vi "IFA300CommandDescriptors.vi"(4 "IFACommand":T2="ReadErrorQueue") -> (0 "Error":bool, 1 "CommandDescriptorOutput":T1={"Command"="ReadErrorQueue", "Mnemonic"="*STAT?", "ActionPath"=["PassCommand", "Communicate", "ParseError", "Done"]})   [LabVIEW 2012]
uses:
  IFA300Command.ctl
  IFA300CommandDescriptor.ctl
  IFA300CommandPhases.ctl
panel:
  in  "CommandDescriptorArray":T1[](array[typedef])=[{"Command"="Reset", "Mnemonic"="*RST", "ActionPath"=["PassCommand", "Communicate", "Done"]}, {"Command"="Version", "Mnemonic"="*IDN?", "ActionPath"=["PassCommand", "Communicate", "Done"]}, {"Command"="ReadErrorQueue", "Mnemonic"="*STAT?", "ActionPath"=["PassCommand", "Communicate", "ParseError", "Done"]}, {"Command"="CountChannels", "Mnemonic"="INST:CNUM?", "ActionPath"=["PassCommand", "Communicate", "ParseNumber", "Done"]}, {"Command"="CheckDaisyChain", "Mnemonic"="INST:IFA? ", "ActionPath"=["PassCommand", "Communicate", "ParseNumber", "Done"]}, {"Command"="MeasureCableResistance", "Mnemonic"="MEAS:RCBL", "ActionPath"=["AddressCommand", "Communicate", "Done"]}, {"Command"="ReadbackCableResistance", "Mnemonic"="READ:RCBL?", "ActionPath"=["PassCommand", "Communicate", "ParseNumber", "Done"]}, {"Command"="MeasureColdResistance", "Mnemonic"="MEAS:RMES", "ActionPath"=["AddressCommand", "Communicate", "Done"]}, {"Command"="ReadbackColdResistance", "Mnemonic"="READ:RMES?", "ActionPath"=["PassCommand", "Communicate", "ParseNumber", "Done"]}, {"Command"="SelectChannel", "Mnemonic"="INST:NSEL", "ActionPath"=["AddressCommand", "Communicate", "Done"]}, {"Command"="MonitorChannel", "Mnemonic"="OUTP:VOLT", "ActionPath"=["AddressCommand", "Communicate", "Done"]}, {"Command"="Complete?", "Mnemonic"="*OPC?", "ActionPath"=["PassCommand", "Communicate", "ParseNumber", "Done"]}, {"Command"="SetHotResistance", "Mnemonic"="CONF:ROP", "ActionPath"=["AppendVariable", "Communicate", "Done"]}, {"Command"="ReadHotResistance", "Mnemonic"="READ:ROP?", "ActionPath"=["PassCommand", "Communicate", "ParseNumber", "Done"]}, {"Command"="ReadAnemometerType", "Mnemonic"="READ:ANEM?", "ActionPath"=["PassCommand", "Communicate", "Done"]}, {"Command"="SetProbeType", "Mnemonic"="CONF:PROB", "ActionPath"=["AppendVariable", "Communicate", "Done"]}, {"Command"="ReadProbeType", "Mnemonic"="READ:PROB?", "ActionPath"=["PassCommand", "Communicate", "Done"]}, {"Command"="SetHighPowerBridgeOn", "Mnemonic"="CONF:HPWR", "ActionPath"=["AppendVariable", "Communicate", "Done"]}, {"Command"="SetCableLength", "Mnemonic"="CONF:CABL", "ActionPath"=["AppendVariable", "Communicate", "Done"]}, {"Command"="RunMode", "Mnemonic"="INIT:STAR", "ActionPath"=["AddressCommand", "Communicate", "Done"]}, {"Command"="StandbyMode", "Mnemonic"="INIT:STOP", "ActionPath"=["AddressCommand", "Communicate", "Done"]}, {"Command"="GetMode", "Mnemonic"="INIT:STAT?", "ActionPath"=["AddressCommand", "Communicate", "ParseNumber", "Done"]}, {"Command"="StandbyAll", "Mnemonic"="ABOR", "ActionPath"=["PassCommand", "Communicate", "Done"]}, {"Command"="OverrideOverheat", "Mnemonic"="CONF:OVHT", "ActionPath"=["AppendVariable", "Communicate", "Done"]}, {"Command"="ReadOverheat", "Mnemonic"="READ:OVHT", "ActionPath"=["PassCommand", "Communicate", "ParseNumber", "Done"]}, {"Command"="ReadBridgeVoltage", "Mnemonic"="READ:BDGV?", "ActionPath"=["PassCommand", "Communicate", "ParseNumber", "Done"]}, {"Command"="SetGain", "Mnemonic"="CONF:GAIN", "ActionPath"=["AppendVariable", "Communicate", "Done"]}, {"Command"="ReadGain", "Mnemonic"="READ:GAIN?", "ActionPath"=["PassCommand", "Communicate", "ParseNumber", "Done"]}, {"Command"="SetOffset", "Mnemonic"="CONF:OFFS", "ActionPath"=["AppendVariable", "Communicate", "Done"]}, {"Command"="ReadOffset", "Mnemonic"="READ:OFFS?", "ActionPath"=["PassCommand", "Communicate", "ParseNumber", "Done"]}, {"Command"="SetLowpassFilter", "Mnemonic"="OUTP:FILT", "ActionPath"=["AppendVariable", "Communicate", "Done"]}, {"Command"="SetHighpassFilter", "Mnemonic"="OUTP:HPAS", "ActionPath"=["AppendVariable", "Communicate", "Done"]}, {"Command"="SetThermocoupleRange", "Mnemonic"="CONF:TEMP", "ActionPath"=["AppendVariable", "Communicate", "Done"]}, {"Command"="MeasureTemperature", "Mnemonic"="MEAS:TEMP", "ActionPath"=["PassCommand", "Communicate", "Done"]}, {"Command"="ReadTemperature", "Mnemonic"="READ:TEMP?", "ActionPath"=["PassCommand", "Communicate", "ParseNumber", "Done"]}, {"Command"="SqWaveFreq", "Mnemonic"="TEST:FREQ", "ActionPath"=["AppendVariable", "Communicate", "Done"]}, {"Command"="SqWaveVolts", "Mnemonic"="TEST:VOLT", "ActionPath"=["AppendVariable", "Communicate", "Done"]}]
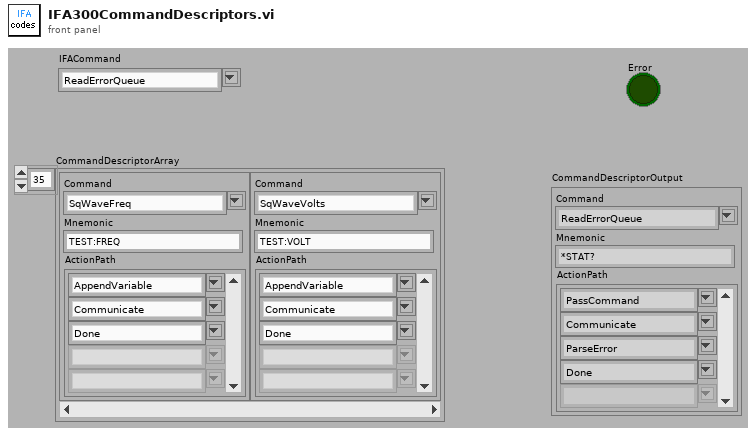
[diagram p1: front panel]
types:
  T1 = typedef "IFA300CommandDescriptor.ctl" = cluster{"Command":T2, "Mnemonic":string, "ActionPath":T3[]}
  T2 = typedef "IFA300Command.ctl" = string
  T3 = typedef "IFA300CommandPhases.ctl" = string
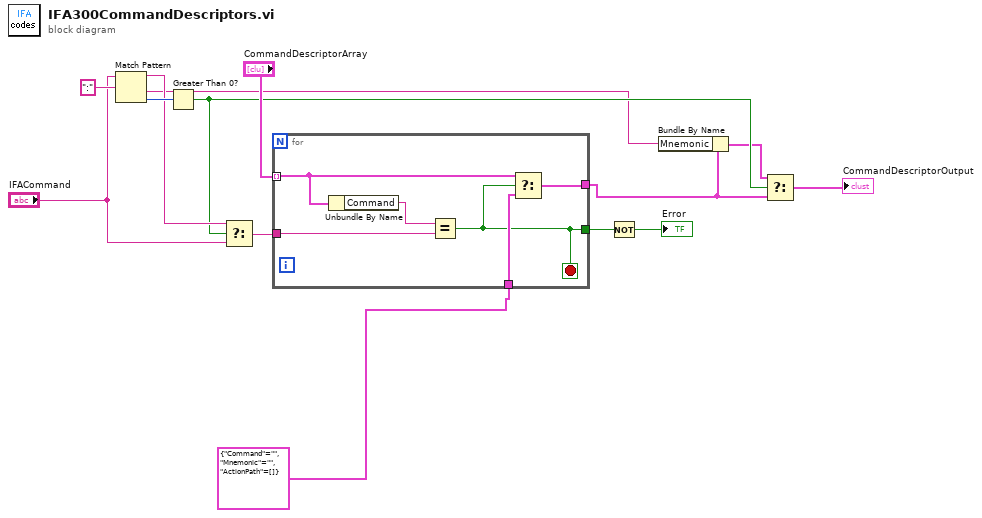
[diagram p0: block diagram]
diagram:
  n1 = Match Pattern(string="IFACommand", regular expression=":") -> (before substring=w7:T2, after substring=w2:T2, offset past match=w10:i32)  [unwired: 2 out]
  n2 = Greater Than 0?(x=w10) -> (x > 0?=w5:bool)
  n3 = Select(t=w7, s=w5, f="IFACommand") -> (s? t:f=w9:T2)
  n4 = for {
    tunnel: "CommandDescriptorArray" -> [w17] mode=indexing
    tunnel: w9 -> [w19]
    tunnel: [w18] -> w4
    tunnel: T1 {"Command"="", "Mnemonic"="", "ActionPath"=[]} ("s? t:f") -> [w16]
    tunnel: [w15] -> w13
    stop <- w15 stop-if-true
    n5 = Unbundle By Name(w17) -> ("Command"=w20:T2)
    n6 = Equal?(x=w20, y=w19) -> (x = y?=w15:bool)
    n7 = Select(t=w17, s=w15, f=w16) -> (s? t:f=w18:T1)
  }
  n8 = Not(x=w13) -> (.not. x?=→"Error":bool)
  n9 = Bundle By Name(cluster=w4, "Mnemonic"=w2) -> (w3:T1)
  n10 = Select(t=w3, s=w5, f=w4) -> (s? t:f=→"CommandDescriptorOutput":T1)
